vi "SiosIfmAngleValue.vi"(1 "Channel 2":i32(knob) scale=1.0..4.0, 2 "Channel 1":i32(knob) scale=1.0..4.0, 3 "Unit":u8(ring) items=["mrad", "seconds"], 4 "Device Number":i32) -> (0 "Angle":dbl)   [LabVIEW 2009]
uses:
  siosifm.dll
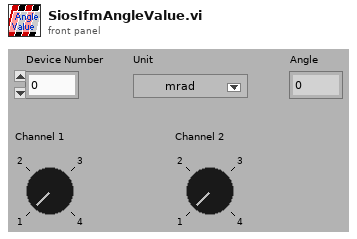
[diagram p1: front panel]
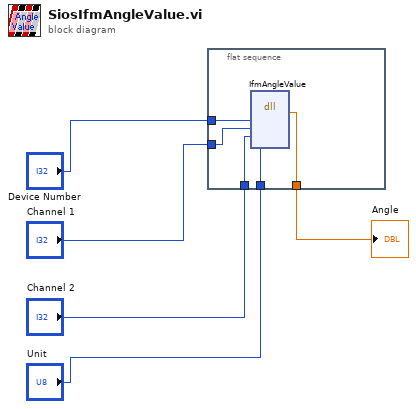
[diagram p0: block diagram]
diagram:
  n1 = flat-sequence {
    tunnel: "Device Number" -> [w10]
    tunnel: "Channel 1" -> [w9]
    tunnel: "Channel 2" -> [w8]
    tunnel: "Unit" -> [w7]
    tunnel: [w6] -> w1
    frame #0 {
      n2 = dll-call lib="C:/WORK/Artem/RE-10/SIOS_IfmDLL/siosifm.dll" fn="IfmAngleValue"("devNumber"=w10, "Channel 1"=w9, "Channel 2"=w8, "Unit"=w7) -> ("angle"=w6:dbl)  [unwired: 7 in, 2 out]
    }
  }
  "Angle" <- w1
